vi "Subtract_Timestamps.vi"(8 "Status/Errors in":refnum<vi>, 9 "Time stamp 2":T1, 10 "Time stamp 1":T1) -> (0 "Status/Errors out":refnum<vi>, 2 "Difference":i32)   [LabVIEW 2010]
uses:
  Controls/GPS_Timestamp.ctl
  Controls/Master.ctl
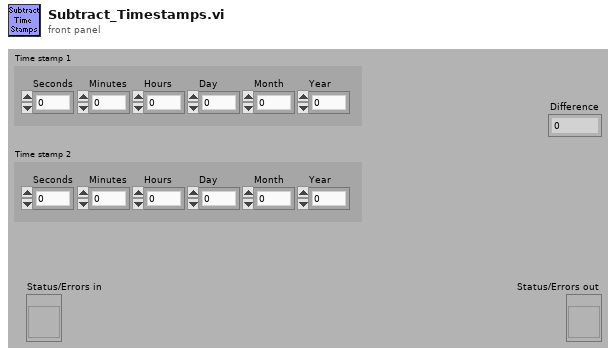
[diagram p1: front panel]
types:
  T1 = typedef "GPS_Timestamp.ctl" = cluster{"Seconds":u8, "Minutes":u8, "Hours":u8, "Day":u8, "Month":u8, "Year":u16}
  T2 = typedef "Comparison_Result.ctl" = enum16{"equal", "1 < 2", "1 > 2", "error in 1", "error in 2", "error in both"}
  T3 = typedef "Master.ctl" = enum16{"Master", "Slave", "General"}
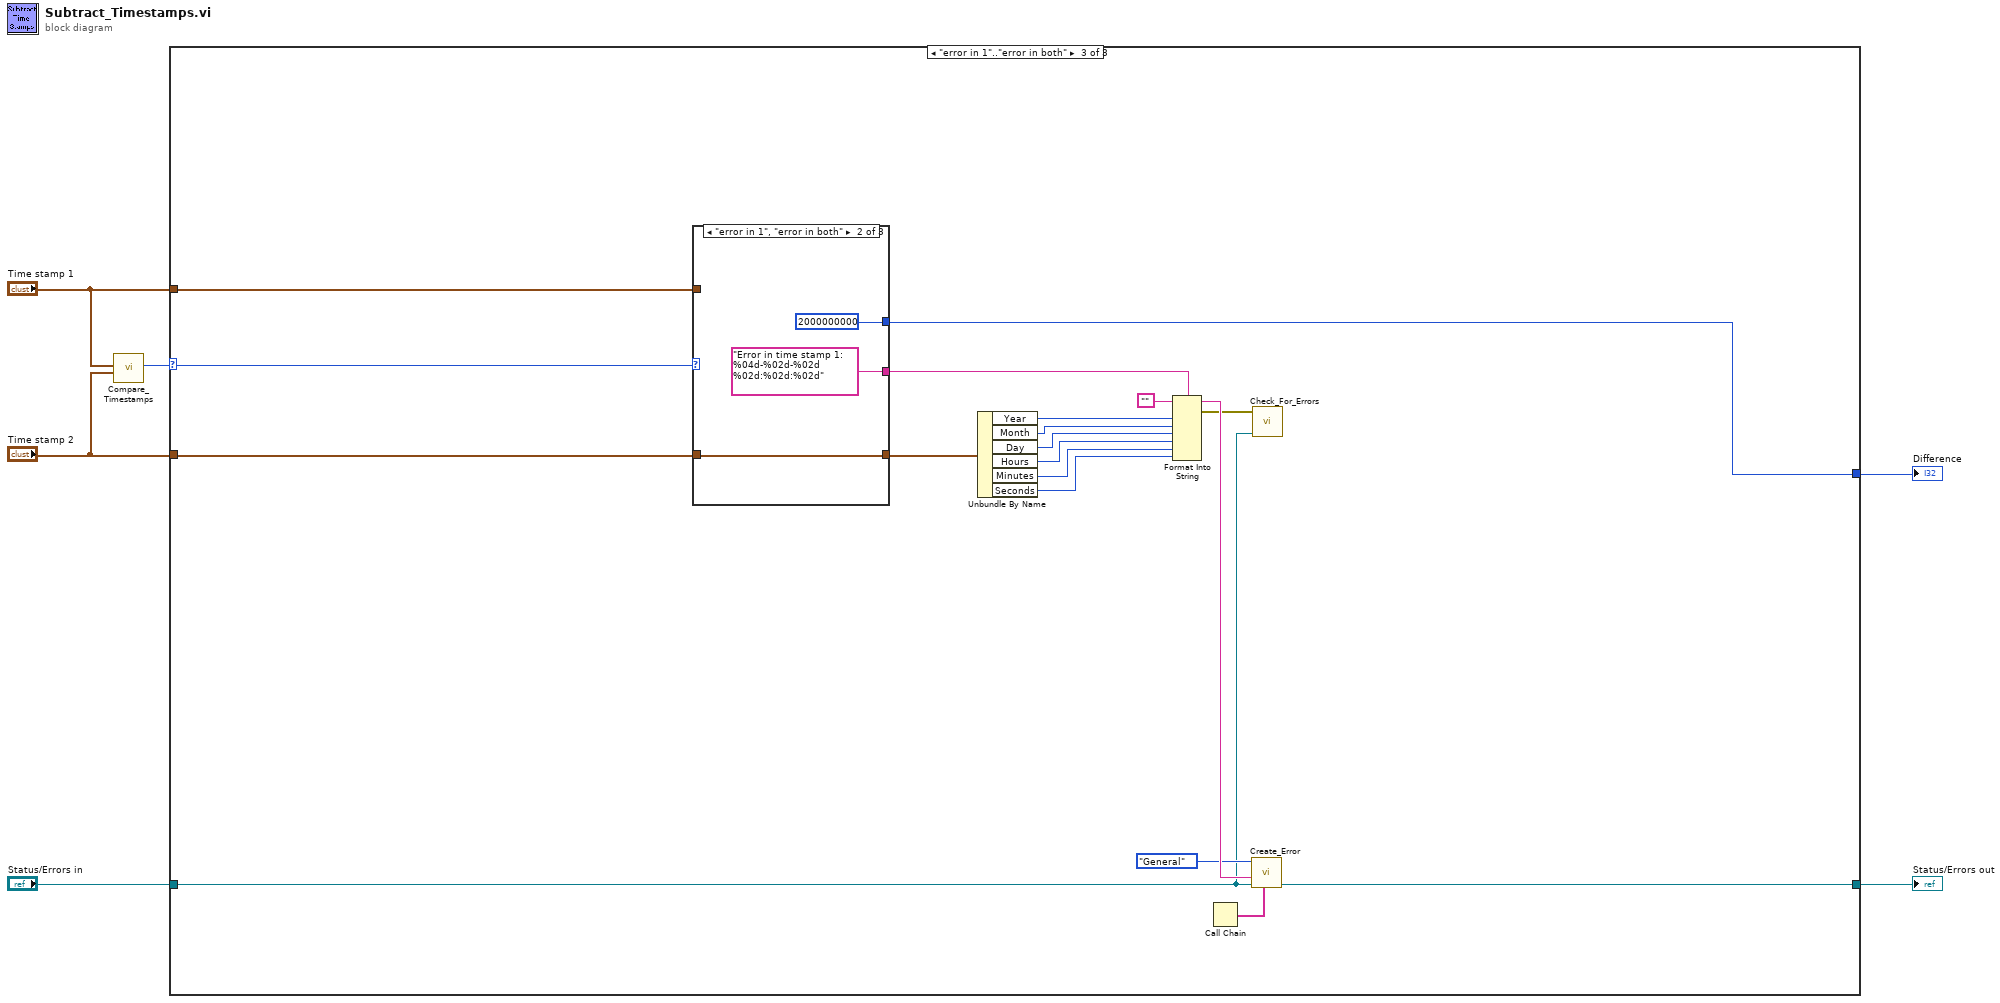
[diagram p0: block diagram]
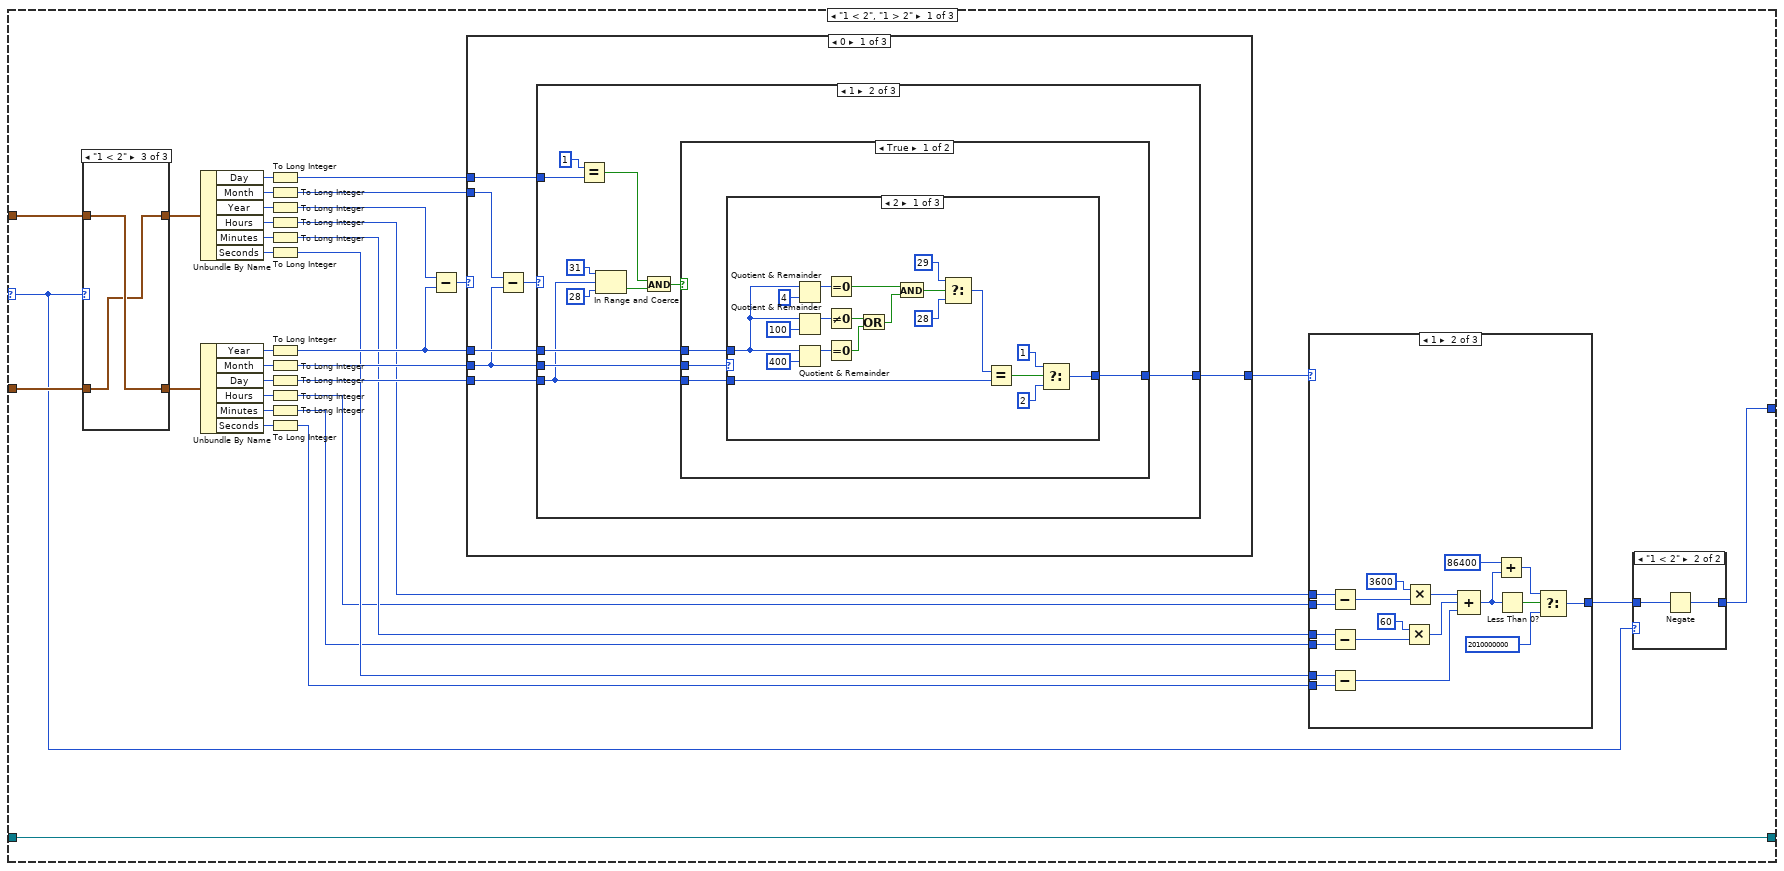
[diagram p2: hidden frame]
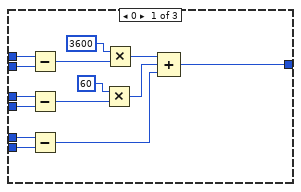
[diagram p4: hidden frame]
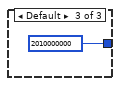
[diagram p5: hidden frame]
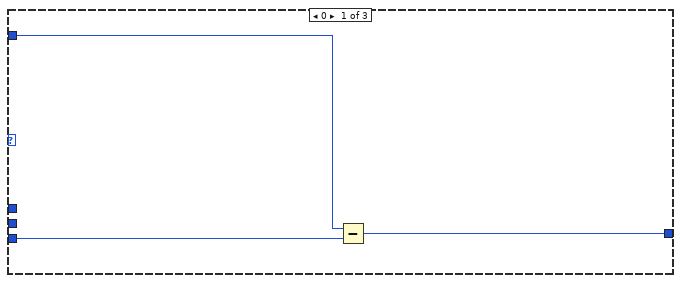
[diagram p6: hidden frame]
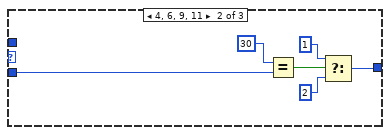
[diagram p7: hidden frame]
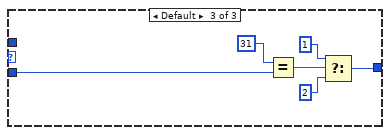
[diagram p8: hidden frame]
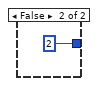
[diagram p9: hidden frame]
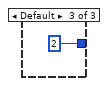
[diagram p10: hidden frame]
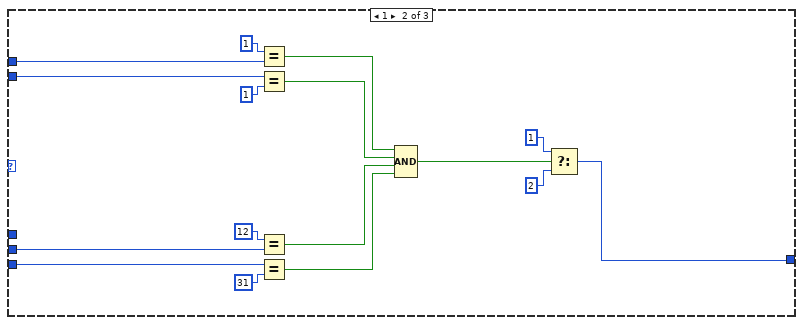
[diagram p11: hidden frame]
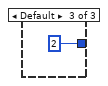
[diagram p12: hidden frame]
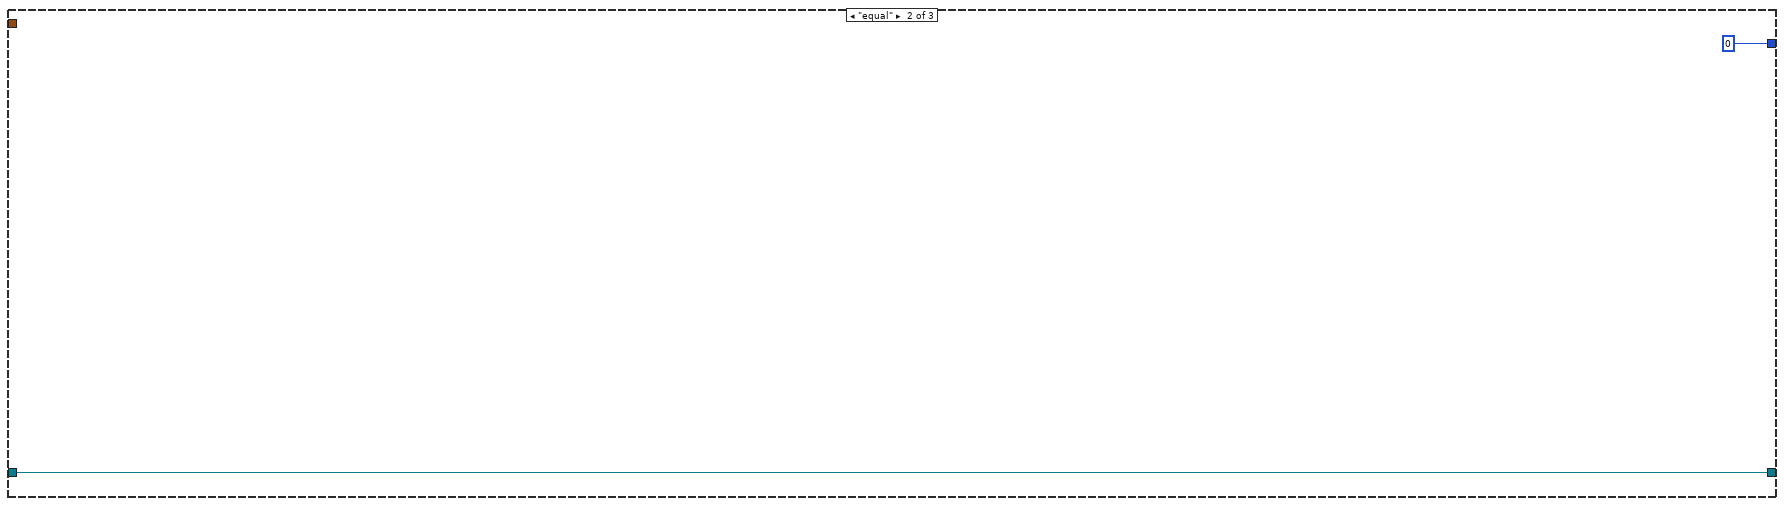
[diagram p15: hidden frame]
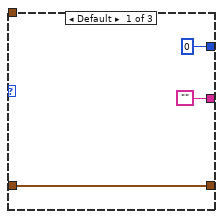
[diagram p16: hidden frame]
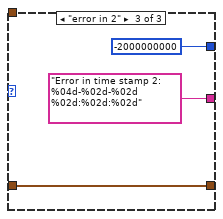
[diagram p17: hidden frame]
diagram:
  n1 = call "Compare_Timestamps.vi"("Time stamp 2"="Time stamp 2", "Time stamp 1"="Time stamp 1") -> ("Comparison result"=w6:T2)  [unwired: 9 out]
  n2 = case shown="\"error in 1\"..\"error in both\"" w6 {
    selector: w6 -> [w10 _ w167]
    tunnel: "Time stamp 1" -> [w40 _ w166]
    tunnel: "Time stamp 2" -> [w39 _ w165]
    tunnel: [w8 0 ("Difference") w163] -> w3
    tunnel: "Status/Errors in" -> [w7 w160 w168]
    tunnel: [w7 w160 w169] -> w1
    frame "1 < 2", "1 > 2" {
      n3 = case shown="\"1 < 2\"" w10 {
        tunnel: w40 -> [w155 w157 w159]
        tunnel: [w155 w157 w158] -> w38
        tunnel: [w154 w156 w159] -> w37
        tunnel: w39 -> [w154 w156 w158]
        frame Default {
        }
        frame "1 > 2" {
        }
        frame "1 < 2" {
        }
      }
      n4 = Unbundle By Name(w38) -> ("Day"=w28:u8, "Month"=w34:u8, "Year"=w36:u16, "Hours"=w14:u8, "Minutes"=w13:u8, "Seconds"=w12:u8)
      n5 = Unbundle By Name(w37) -> ("Year"=w35:u16, "Month"=w33:u8, "Day"=w32:u8, "Hours"=w31:u8, "Minutes"=w30:u8, "Seconds"=w29:u8)
      n6 = To Long Integer(number=w28) -> (32bit integer=w26:i32)
      n7 = To Long Integer(number=w34) -> (32bit integer=w25:i32)
      n8 = To Long Integer(number=w36) -> (32bit integer=w24:i32)
      n9 = To Long Integer(number=w14) -> (32bit integer=w20:i32)
      n10 = To Long Integer(number=w13) -> (32bit integer=w19:i32)
      n11 = To Long Integer(number=w12) -> (32bit integer=w18:i32)
      n12 = To Long Integer(number=w35) -> (32bit integer=w21:i32)
      n13 = To Long Integer(number=w33) -> (32bit integer=w22:i32)
      n14 = To Long Integer(number=w32) -> (32bit integer=w23:i32)
      n15 = To Long Integer(number=w31) -> (32bit integer=w17:i32)
      n16 = To Long Integer(number=w30) -> (32bit integer=w16:i32)
      n17 = To Long Integer(number=w29) -> (32bit integer=w15:i32)
      n18 = Subtract(x=w24, y=w21) -> (x-y=w27:i32)
      n19 = case shown="0" w27 {
        tunnel: w26 -> [w82 w142 _]
        tunnel: w25 -> [w84 w149 _]
        tunnel: w23 -> [w81 w146 _]
        tunnel: w22 -> [w79 w145 _]
        tunnel: w21 -> [w80 _ _]
        tunnel: [w78 w150 2 ("t")] -> w11
        frame 0 {
          n20 = Subtract(x=w84, y=w79) -> (x-y=w83:i32)
          n21 = case shown="1" w83 {
            tunnel: w82 -> [w87 w97 _]
            tunnel: w81 -> [w86 w89 _]
            tunnel: w80 -> [_ w98 _]
            tunnel: w79 -> [_ w90 _]
            tunnel: [w85 w88 2 ("t")] -> w78
            frame 0 {
              n22 = Subtract(x=w87, y=w86) -> (x-y=w85:i32)
            }
            frame 1 {
              n23 = Equal?(x=1, y=w97) -> (x = y?=w92:bool)
              n24 = In Range and Coerce(upper limit=31, x=w89, lower limit=28) -> (In Range?=w91:bool)  [unwired: 1 out]
              n25 = And(x=w92, y=w91) -> (x .and. y?=w93:bool)
              n26 = case shown="True" w93 {
                tunnel: w98 -> [w101 _]
                tunnel: w90 -> [w102 _]
                tunnel: w89 -> [w100 _]
                tunnel: [w99 2 ("t")] -> w88
                frame True {
                  n27 = case shown="2" w102 {
                    tunnel: w101 -> [w119 _ _]
                    tunnel: w100 -> [w111 w128 w134]
                    tunnel: [w103 w124 w130] -> w99
                    frame 2 {
                      n28 = Quotient & Remainder(x=w119, y=4) -> (x-y*floor(x/y)=w116:i32)  [unwired: 1 out]
                      n29 = Quotient & Remainder(x=w119, y=100) -> (x-y*floor(x/y)=w118:i32)  [unwired: 1 out]
                      n30 = Quotient & Remainder(x=w119, y=400) -> (x-y*floor(x/y)=w117:i32)  [unwired: 1 out]
                      n31 = Equal To 0?(x=w116) -> (x = 0?=w112:bool)
                      n32 = Not Equal To 0?(x=w118) -> (x != 0?=w115:bool)
                      n33 = Equal To 0?(x=w117) -> (x = 0?=w114:bool)
                      n34 = Or(x=w115, y=w114) -> (x .or. y?=w113:bool)
                      n35 = And(x=w112, y=w113) -> (x .and. y?=w110:bool)
                      n36 = Select(t=29 ("x"), s=w110, f=28 ("x")) -> (s? t:f=w107:i32)
                      n37 = Equal?(x=w107, y=w111) -> (x = y?=w106:bool)
                      n38 = Select(t=1, s=w106, f=2 ("t")) -> (s? t:f=w103:i32)
                    }
                    frame 4, 6, 9, 11 {
                      n39 = Equal?(x=30, y=w128) -> (x = y?=w127:bool)
                      n40 = Select(t=1, s=w127, f=2 ("t")) -> (s? t:f=w124:i32)
                    }
                    frame Default {
                      n41 = Equal?(x=31, y=w134) -> (x = y?=w133:bool)
                      n42 = Select(t=1, s=w133, f=2 ("t")) -> (s? t:f=w130:i32)
                    }
                  }
                }
                frame False {
                }
              }
            }
            frame Default {
            }
          }
        }
        frame 1 {
          n43 = Equal?(x=1, y=w142) -> (x = y?=w141:bool)
          n44 = Equal?(x=w149, y=1) -> (x = y?=w140:bool)
          n45 = Equal?(x=12, y=w145) -> (x = y?=w138:bool)
          n46 = Equal?(x=w146, y=31) -> (x = y?=w139:bool)
          n47 = Compound Arithmetic op=AND(w141, w140, w138, w139) -> (w137:bool)
          n48 = Select(t=1, s=w137, f=2 ("t")) -> (s? t:f=w150:i32)
        }
        frame Default {
        }
      }
      n49 = case shown="1" w11 {
        tunnel: w17 -> [w56 w75 _]
        tunnel: w16 -> [w52 w71 _]
        tunnel: w15 -> [w50 w69 _]
        tunnel: w20 -> [w57 w76 _]
        tunnel: w19 -> [w53 w72 _]
        tunnel: w18 -> [w51 w70 _]
        tunnel: [w44 w58 2010000000 ("Difference")] -> w9
        frame 0 {
          n50 = Subtract(x=w57, y=w56) -> (x-y=w55:i32)
          n51 = Subtract(x=w53, y=w52) -> (x-y=w48:i32)
          n52 = Subtract(x=w51, y=w50) -> (x-y=w45:i32)
          n53 = Multiply(x=60, y=w48) -> (x*y=w46:i32)
          n54 = Multiply(x=3600, y=w55) -> (x*y=w47:i32)
          n55 = Compound Arithmetic op=ADD(w47, w46, w45) -> (w44:i32)
        }
        frame 1 {
          n56 = Subtract(x=w76, y=w75) -> (x-y=w74:i32)
          n57 = Subtract(x=w72, y=w71) -> (x-y=w67:i32)
          n58 = Subtract(x=w70, y=w69) -> (x-y=w64:i32)
          n59 = Multiply(x=60, y=w67) -> (x*y=w65:i32)
          n60 = Multiply(x=3600, y=w74) -> (x*y=w66:i32)
          n61 = Compound Arithmetic op=ADD(w66, w65, w64) -> (w61:i32)
          n62 = Add(x=86400, y=w61) -> (x+y=w62:i32)
          n63 = Less Than 0?(x=w61) -> (x < 0?=w63:bool)
          n64 = Select(t=w62, s=w63, f=2010000000 ("Difference")) -> (s? t:f=w58:i32)
        }
        frame Default {
        }
      }
      n65 = case shown="\"1 < 2\"" w10 {
        tunnel: w9 -> [w41 w43]
        tunnel: [w41 w42] -> w8
        frame Default {
        }
        frame "1 < 2" {
          n66 = Negate(x=w43) -> (-x=w42:i32)
        }
      }
    }
    frame "equal" {
    }
    frame "error in 1".."error in both" {
      n67 = case shown="\"error in 1\", \"error in both\"" w167 {
        tunnel: w166 -> [_ _ _]
        tunnel: w165 -> [w183 w186 w189]
        tunnel: [w183 w186 w189] -> w164
        tunnel: [0 ("Difference") 2000000000 ("Difference") -2000000000 ("Difference")] -> w163
        tunnel: ["" "Error in time stamp 1: %04d-%02d-%02d %02d:%02d:%02d" ("format string") "Error in time stamp 2: %04d-%02d-%02d %02d:%02d:%02d" ("format string")] -> w162
        frame Default {
        }
        frame "error in 1", "error in both" {
        }
        frame "error in 2" {
        }
      }
      n68 = Unbundle By Name(w164) -> ("Year"=w178:u16, "Month"=w177:u8, "Day"=w176:u8, "Hours"=w175:u8, "Minutes"=w174:u8, "Seconds"=w173:u8)
      n69 = Format Into String(format string=w162, initial string="", w178, w177, w176, w175, w174, w173) -> (resulting string=w172:string, error out=w171:errorcluster)  [unwired: 1 in]
      n70 = Call Chain() -> (call chain=w180:string[])
      n71 = call "Create_Error.vi"("Call chain"=w180, "Status/Errors in"=w168, "HiSPARC error"=w172, "Master?"=Master."General") -> ("Status/Errors out"=w169:refnum<vi>)  [unwired: 2 in, 5 out]
      n72 = call "Check_For_Errors.vi"("Status/Errors in"=w168, "error in"=w171) -> ()  [unwired: 10 out]
    }
  }
  "Difference" <- w3
  "Status/Errors out" <- w1
